vi "压装试验判定.vi"(7 "Result":refnum<vi>, 10 "判定参数":T1, 11 "XY曲线":cluster{"X":dbl[], "Y":dbl[]}[](array[cluster])) -> (2 "判定项长度":i32, 3 "OK？":bool)   [LabVIEW 2020]
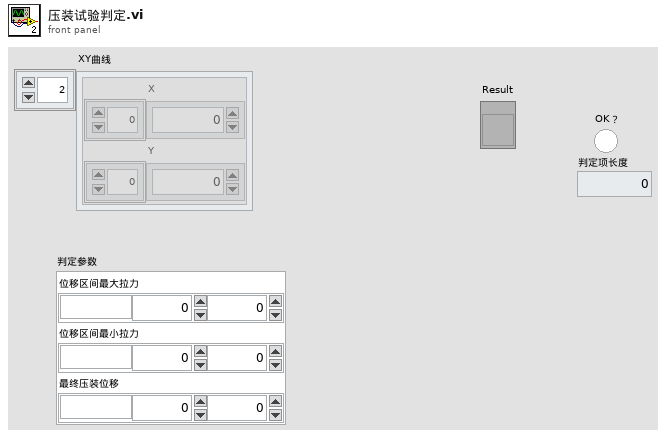
[diagram p1: front panel]
types:
  T1 = cluster{"位移区间最大拉力":cluster{"单位":string, "下限":dbl, "上限":dbl}, "位移区间最小拉力":cluster{"单位":string, "下限":dbl, "上限":dbl}, "最终压装位移":cluster{"单位":string, "下限":dbl, "上限":dbl}}
  T2 = cluster{"1位移":cluster{"单位":string, "下限":dbl, "上限":dbl}, "1压力":cluster{"单位":string, "下限":dbl, "上限":dbl}}
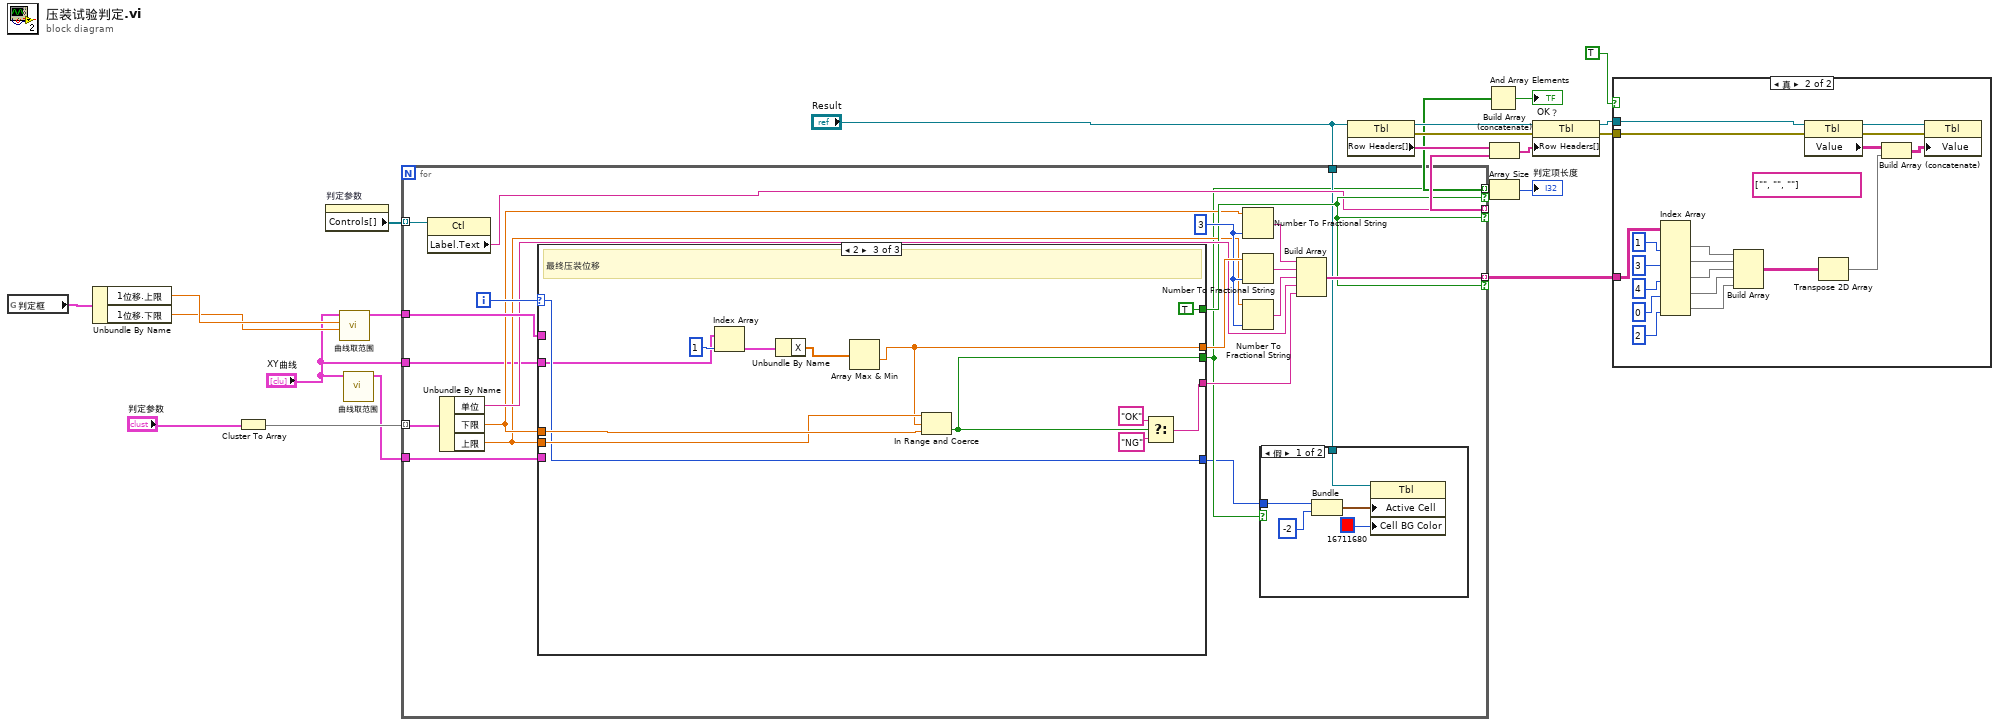
[diagram p0: block diagram]
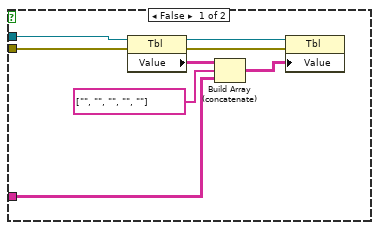
[diagram p2: hidden frame]
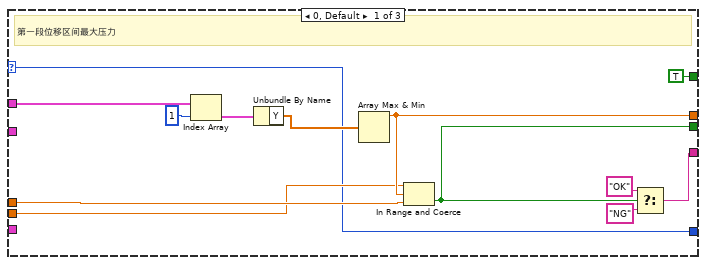
[diagram p4: hidden frame]
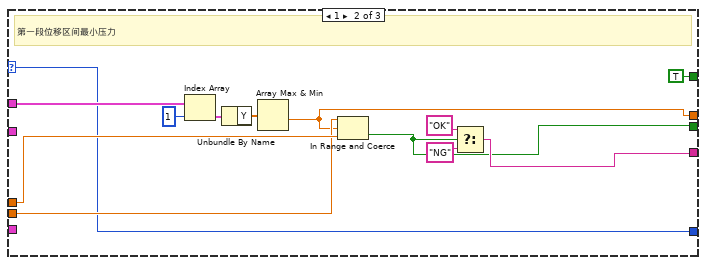
[diagram p5: hidden frame]
diagram:
  n1 = global read "判定参数.vi" "判定框"() -> (w4:T2)
  n2 = Unbundle By Name(w4) -> ("1位移.上限"=w6:dbl, "1位移.下限"=w5:dbl)
  n3 = Cluster To Array(cluster="判定参数") -> (array=w22:cluster{"单位":string, "下限":dbl, "上限":dbl}[])
  n4 = property on="判定参数" class="Clust (严格)"() -> ("Controls[]"=w12:refnum<vi>[])  [unwired: 2 in, 2 out]
  n5 = call "曲线取范围.vi"("下限"=w5, "上限"=w6, "曲线In"="XY曲线") -> ("曲线Out"=w8:cluster{"X":dbl[], "Y":dbl[]}[])  [unwired: 8 in]
  n6 = call "曲线取范围.vi"("曲线In"="XY曲线") -> ("曲线Out"=w2:cluster{"X":dbl[], "Y":dbl[]}[])  [unwired: 10 in]
  n7 = for {
    tunnel: w22 -> [w43] mode=indexing
    tunnel: w12 -> [w41] mode=indexing
    tunnel: w8 -> [w39]
    tunnel: [w24] -> w10 mode=indexing if=w31
    tunnel: [w32] -> w13 mode=indexing if=w31
    tunnel: [w28] -> w15 mode=indexing if=w31
    tunnel: "XY曲线" -> [w27]
    tunnel: w2 -> [w26]
    tunnel: "Result" -> [w25]
    i -> [w42]
    w38 = i16 3 ("精度(6)")
    n8 = property class="Ctl"(reference=w41) -> ("Label.Text"=w28:string)  [unwired: 1 in, 2 out]
    n9 = Unbundle By Name(w43) -> ("单位"=w33:string, "下限"=w30:dbl, "上限"=w29:dbl)
    n10 = case shown="2" w42 {
      selector: w42 -> [w49 w62 w79]
      tunnel: [w58 w65 w78] -> w40
      tunnel: w39 -> [w61 w74 _]
      tunnel: [w55 w70 w84] -> w34
      tunnel: [w54 w69 w83] -> w24
      tunnel: w30 -> [w53 w68 w82]
      tunnel: w29 -> [w52 w67 w81]
      tunnel: [TRUE TRUE TRUE] -> w31
      tunnel: w27 -> [_ _ w77]
      tunnel: w26 -> [_ _ _]
      tunnel: [w49 w62 w79] -> w23
      frame 0, Default {
        # "第一段位移区间最大压力"
        n11 = Index Array(array=w61, index=1 ("索引")) -> (element=w59:cluster{"X":dbl[], "Y":dbl[]})
        n12 = Unbundle By Name(w59) -> ("Y"=w50:dbl[])
        n13 = Array Max & Min(array=w50) -> (max value=w58:dbl)  [unwired: 3 out]
        n14 = In Range and Coerce(upper limit=w52, x=w58, lower limit=w53) -> (In Range?=w54:bool)  [unwired: 1 out]
        n15 = Select(t="OK", s=w54, f="NG") -> (s? t:f=w55:string)
      }
      frame 1 {
        # "第一段位移区间最小压力"
        n16 = Index Array(array=w74, index=1 ("索引")) -> (element=w73:cluster{"X":dbl[], "Y":dbl[]})
        n17 = Unbundle By Name(w73) -> ("Y"=w64:dbl[])
        n18 = Array Max & Min(array=w64) -> (min value=w65:dbl)  [unwired: 3 out]
        n19 = In Range and Coerce(upper limit=w67, x=w65, lower limit=w68) -> (In Range?=w69:bool)  [unwired: 1 out]
        n20 = Select(t="OK", s=w69, f="NG") -> (s? t:f=w70:string)
      }
      frame 2 {
        # "最终压装位移"
        n21 = Index Array(array=w77, index=1 ("索引")) -> (element=w76:cluster{"X":dbl[], "Y":dbl[]})
        n22 = Unbundle By Name(w76) -> ("X"=w75:dbl[])
        n23 = Array Max & Min(array=w75) -> (min value=w78:dbl)  [unwired: 3 out]
        n24 = In Range and Coerce(upper limit=w81, x=w78, lower limit=w82) -> (In Range?=w83:bool)  [unwired: 1 out]
        n25 = Select(t="OK", s=w83, f="NG") -> (s? t:f=w84:string)
      }
    }
    n26 = Number To Fractional String(number=w30, precision (6)=w38) -> (F-format string=w37:string)  [unwired: 2 in]
    n27 = Number To Fractional String(number=w40, precision (6)=w38) -> (F-format string=w36:string)  [unwired: 2 in]
    n28 = Number To Fractional String(number=w29, precision (6)=w38) -> (F-format string=w35:string)  [unwired: 2 in]
    n29 = case shown="假" w24 {
      tunnel: w25 -> [w48 _]
      tunnel: w23 -> [w44 _]
      frame False {
        n30 = Bundle(w44, "索引"=-2) -> (w45:cluster{i32, "索引":i32})  [unwired: 1 in]
        n31 = property class="Tbl"(reference=w48, "Active Cell"=w45, "Cell BG Color"=u32 16711680 ("活动单元格:单元格背景色")) -> ()  [unwired: 1 in, 2 out]
      }
      frame True {
      }
    }
    n32 = Build Array(w37, w36, w35, w33, w34) -> (w32:string[])
  }
  n33 = property class="Tbl"(reference="Result") -> (reference out=w17:refnum<vi>, error out=w20:errorcluster, "Row Headers[]"=w14:string[])  [unwired: 1 in]
  n34 = And Array Elements(Boolean array=w10) -> (logical AND=→"OK？":bool)
  n35 = Build Array (concatenate)(w14, w15) -> (w16:string[])
  n36 = Array Size(array=w10) -> (size(s)=→"判定项长度":i32)
  n37 = property class="Tbl"(reference=w17, error in=w20, "Row Headers[]"=w16) -> (reference out=w18:refnum<vi>, error out=w19:errorcluster)
  n38 = case shown="真" TRUE {
    tunnel: w19 -> [w93 w112]
    tunnel: w18 -> [w90 w109]
    tunnel: w13 -> [w89 w108]
    frame False {
      n39 = property class="Tbl"(reference=w90, error in=w93) -> (reference out=w91:refnum<vi>, error out=w92:errorcluster, "Value"=w94:string[][])
      n40 = Build Array (concatenate)(w94, string[] ["", "", "", "", ""], w89) -> (w95:string[][])
      n41 = property class="Tbl"(reference=w91, error in=w92, "Value"=w95) -> ()  [unwired: 2 out]
    }
    frame True {
      (unwired) string[] ["", "", ""]
      n42 = Index Array(array=w108, index (col) #1=1 ("禁用的索引 (列)"), index (col) #2=3 ("索引 (列)"), index (col) #3=4 ("索引 (列)"), index (col) #4=0 ("索引 (列)"), index (col) #5=2 ("索引 (列)")) -> (element #1=w104:string[], element #2=w103:string[], element #3=w102:string[], element #4=w97:string[], element #5=w96:string[])  [unwired: 5 in]
      n43 = Build Array(w104, w103, w102, w97, w96) -> (w101:string[][])
      n44 = property class="Tbl"(reference=w109, error in=w112) -> (reference out=w110:refnum<vi>, error out=w111:errorcluster, "Value"=w113:string[][])
      n45 = Transpose 2D Array(2D array=w101) -> (transposed array=w100:string[][])
      n46 = Build Array (concatenate)(w113, w100) -> (w114:string[][])
      n47 = property class="Tbl"(reference=w110, error in=w111, "Value"=w114) -> ()  [unwired: 2 out]
    }
  }
